vi "Monitor Date.vi"(8 "error in (no error)":errorcluster, 10 "Address (0)":i32, 11 "VISA resource name":refnum<visa-resource-name>) -> (0 "error out":errorcluster, 1 "Day":i32, 2 "Month":i32, 3 "VISA resource name out":refnum<visa-resource-name>, 5 "Year":i32)   [LabVIEW 2016, in "Environment Chamber.lvlib" / "Climatic Chamber.lvlib"]
doc: "<b>Date monitor</b>\n\nReturns the date of the internal calendar."
uses:
  Climatic Chamber.lvlib
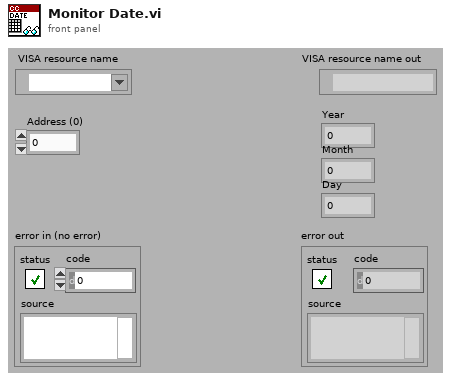
[diagram p1: front panel]
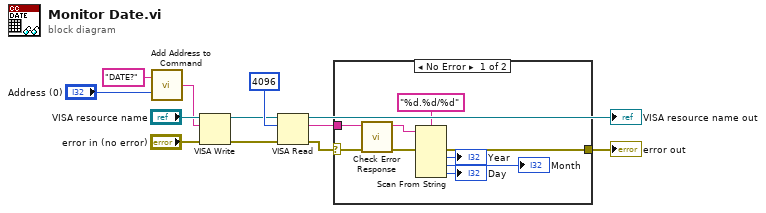
[diagram p0: block diagram]
diagram:
  n1 = call "Add Address to Command.vi"("Address (0)"="Address (0)", "Command"="DATE?") -> ("Command OUT"=w5:string)
  n2 = VISA Write(VISA resource name="VISA resource name", write buffer=w5, error in (no error)="error in (no error)") -> (VISA resource name out=w9:refnum<visa-resource-name>, error out=w8:errorcluster)  [unwired: 1 out]
  n3 = VISA Read(VISA resource name=w9, byte count=u32 4096, error in (no error)=w8) -> (VISA resource name out=→"VISA resource name out":refnum<visa-resource-name>, read buffer=w3:string, error out=w4:errorcluster)  [unwired: 1 out]
  n4 = case shown="No Error" w4 {
    selector: w4 -> [w20 w22]
    tunnel: w3 -> [w21 _]
    tunnel: [w17 w22] -> w2
    frame No Error {
      n5 = call "Check Error Response.vi"("error in (no error)"=w20, "read String"=w21) -> ("error out"=w19:errorcluster, "String out"=w18:string)  [unwired: 7 in, 1 out]
      n6 = Scan From String(format string="%d.%d/%d", input string=w18, error in=w19) -> (error out=w17:errorcluster, output 1=→"Year":i32, output 2=→"Month":i32, output 3=→"Day":i32)  [unwired: 4 in, 2 out]
    }
    frame Error {
    }
  }
  "error out" <- w2
